vi "Client Cancel Call Context.vi"(8 "error in":errorcluster, 11 "Context ID in":T1) -> (0 "error out":errorcluster, 3 "Context ID out":T1)   [LabVIEW 2019, in "grpc-lvsupport.lvlib"]
uses:
  grpc-lvsupport.lvlib
  grpcId.ctl
  <vilib>/Utility/file.llb/Application Directory.vi
  <vilib>/Utility/error.llb/Error Cluster From Error Code.vi
  <resource>/labview_grpc_server.dll
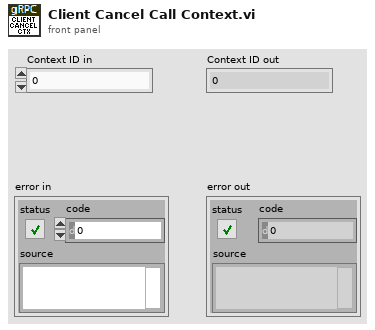
[diagram p1: front panel]
types:
  T1 = typedef "grpc-lvsupport.lvlib/grpcId.ctl" = u64
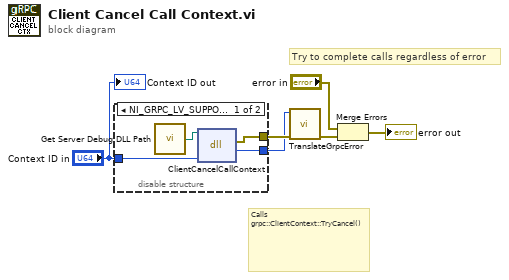
[diagram p0: block diagram]
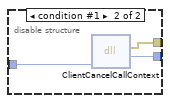
[diagram p2: hidden frame]
diagram:
  # "Calls \ngrpc::ClientContext::TryCancel()"
  # "Try to complete calls regardless of error"
  n1 = disable-structure shown="NI_GRPC_LV_SUPPORT_DEBUG==True&&RUN_TIME_ENGINE==False" {
    disable-tunnel: [w10 w13] -> w6
    disable-tunnel: "Context ID in" -> [w9 w12]
    disable-tunnel: [w7 w11] -> w5
    frame condition #0 (active) {
      n2 = call "Get Server Debug DLL Path.vi"() -> ("DLL Path"=w8:path)
      n3 = dll-call lib="?" fn="ClientCancelCallContext"(path in=w8, "contextId"=w9) -> (error out=w10:errorcluster, "return type"=w7:i32)  [unwired: 3 in, 1 out]
    }
    frame condition #1 {
      n4 = dll-call lib="C:/Program Files (x86)/National Instruments/LabVIEW 2024/resource/labview_grpc_server.*" fn="ClientCancelCallContext"("contextId"=w12) -> (error out=w13:errorcluster, "return type"=w11:i32)  [unwired: 4 in, 1 out]
    }
  }
  n5 = call "TranslateGrpcError.vi"("error in"=w6, "Error Code"=w5) -> ("error out"=w4:errorcluster)  [unwired: 9 in]
  n6 = Merge Errors("error in", w4) -> (→"error out":errorcluster)
  "Context ID out" <- "Context ID in"
